vi "write out sonde row.vi"(0 "NI_report in":refnum<class "NI_report.lvclass">, 2 "Columns":i32[](array[numeric]), 3 "Column of Volume":i32, 5 "Sample Sheet Data Row Cluster":T1={"Head\nPressure"=0.0, "Depth"=0.0, "comment "="", "Sonde Data Cluster"={"Cumulative\nVolume (ml)"=100.0, "Specific\nCond (mS)"=2.0, "Dissolved\nOxygen mg/L"=3.0, "pH"=4.0, "ORP"=5.0, "Temp deg C"=26.0, "Salinity"=7.0}, "Aux1"=0.0, "Aux2"=0.0, "Aux3"=0.0} {"Sonde Data Cluster"."Salinity" format="%_3g"; "Sonde Data Cluster"."Temp deg C" format="%_2g"; "Sonde Data Cluster"."ORP" format="%_4g"; "Sonde Data Cluster"."pH" format="%_4g"; "Sonde Data Cluster"."Dissolved\nOxygen mg/L" format="%_4g"; "Sonde Data Cluster"."Specific\nCond (mS)" format="%_4g"; "Sonde Data Cluster"."Cumulative\nVolume (ml)" format="%#_4g"}, 9 "row index":i32, 11 "error in (no error)":errorcluster, 13 "start of last occupied row":cluster{"row":i32, "column":i32}) -> (4 "NI_report out":refnum<class "NI_report.lvclass">, 14 "row index out":i32, 15 "error out":errorcluster)   [LabVIEW 2016]
uses:
  <vilib>/Utility/NIReport.llb/NI_report.lvclass
  sample data row cluster.ctl
  sonde cluster.ctl
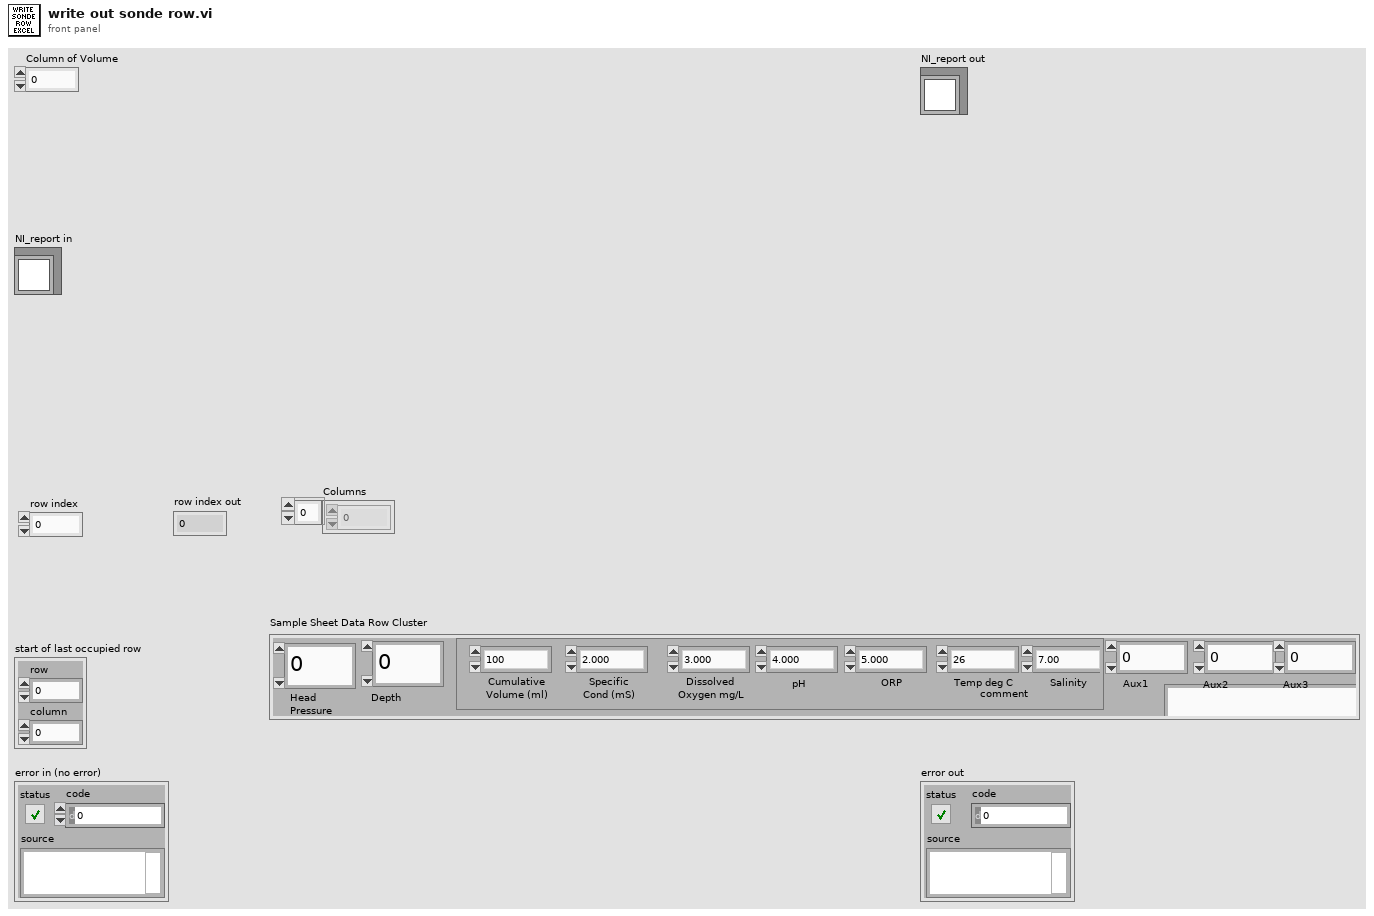
[diagram p1: front panel]
types:
  T1 = typedef "sample data row cluster.ctl" = cluster{"Head\nPressure":dbl, "Depth":dbl, "comment ":string, "Sonde Data Cluster":T2, "Aux1":dbl, "Aux2":dbl, "Aux3":dbl}
  T2 = typedef "sonde cluster.ctl" = cluster{"Cumulative\nVolume (ml)":dbl, "Specific\nCond (mS)":dbl, "Dissolved\nOxygen mg/L":dbl, "pH":dbl, "ORP":dbl, "Temp deg C":dbl, "Salinity":dbl}
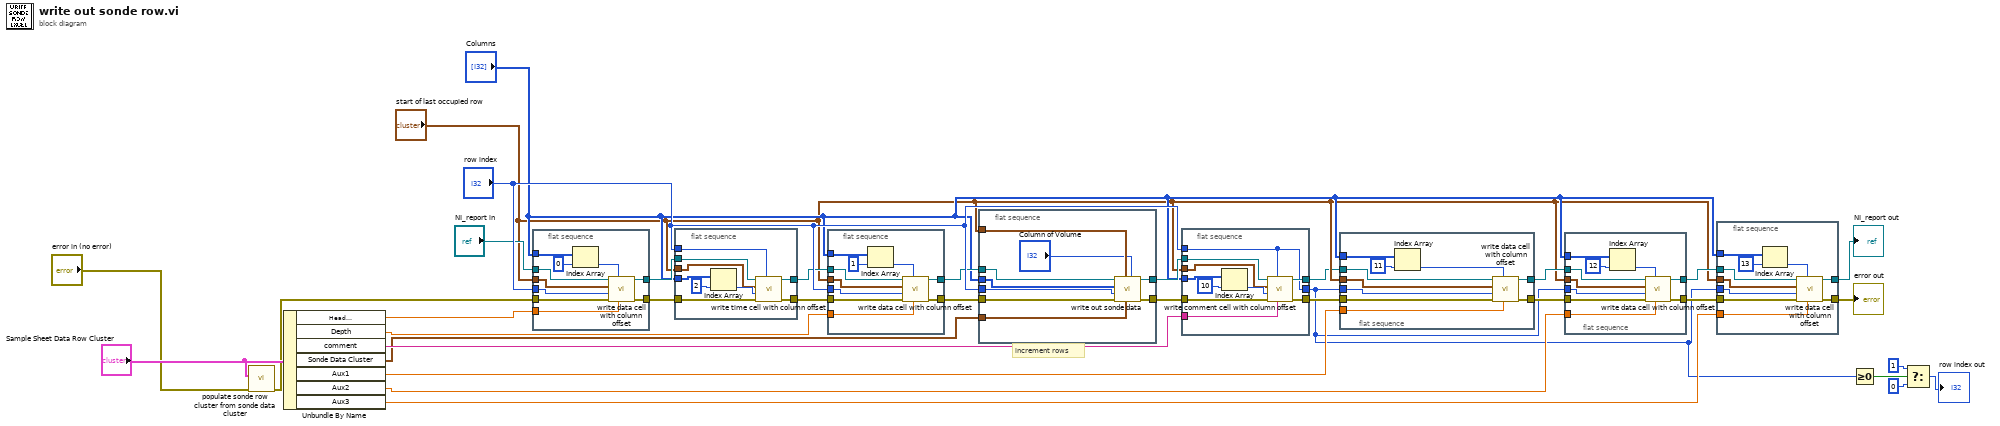
[diagram p0: block diagram]
diagram:
  # "increment rows"
  n1 = call "populate sonde row cluster from sonde data cluster.vi"("error in (no error)"="error in (no error)", "Sample Sheet Data Row Cluster"="Sample Sheet Data Row Cluster") -> ("error out"=w1:errorcluster)  [unwired: 7 in, 2 out]
  n2 = Unbundle By Name("Sample Sheet Data Row Cluster") -> ("Head\nPressure"=w25:dbl, "Depth"=w24:dbl, "comment"=w23:string, "Sonde Data Cluster"=w22:T2, "Aux1"=w16:dbl, "Aux2"=w5:dbl, "Aux3"=w4:dbl)
  n3 = flat-sequence {
    tunnel: "row index" -> [w45]
    tunnel: "start of last occupied row" -> [w44]
    tunnel: [w42] -> w31
    tunnel: [w41] -> w30
    tunnel: "NI_report in" -> [w39]
    tunnel: w1 -> [w38]
    tunnel: "Columns" -> [w37]
    tunnel: w25 -> [w36]
    frame #0 {
      n4 = Index Array(array=w37, index=0) -> (element=w43:i32)
      n5 = call "write data cell with column offset.vi"("Data Input"=w36, "data column"=w43, "error in (no error)"=w38, "row offset"=w45, "start of last occupied row"=w44, "NI_report in"=w39) -> ("error out"=w42:errorcluster, "NI_report out"=w41:refnum<class "NI_report.lvclass">)  [unwired: 4 in]
    }
  }
  n6 = flat-sequence {
    tunnel: "row index" -> [w54]
    tunnel: "start of last occupied row" -> [w51]
    tunnel: w31 -> [w50]
    tunnel: w30 -> [w49]
    tunnel: [w48] -> w29
    tunnel: [w47] -> w28
    tunnel: "Columns" -> [w46]
    frame #0 {
      n7 = Index Array(array=w46, index=2) -> (element=w53:i32)
      n8 = call "write time cell with column offset.vi"("Header offset"=w54, "error in (no error)"=w50, "time column offset"=w53, "start of last occupied row"=w51, "NI_report in"=w49) -> ("error out"=w47:errorcluster, "NI_report out"=w48:refnum<class "NI_report.lvclass">)  [unwired: 5 in]
    }
  }
  n9 = flat-sequence {
    tunnel: "row index" -> [w64]
    tunnel: [w63] -> w34
    tunnel: "start of last occupied row" -> [w62]
    tunnel: w29 -> [w61]
    tunnel: w28 -> [w60]
    tunnel: [w59] -> w27
    tunnel: "Columns" -> [w58]
    tunnel: w24 -> [w55]
    frame #0 {
      n10 = Index Array(array=w58, index=1) -> (element=w56:i32)
      n11 = call "write data cell with column offset.vi"("Data Input"=w55, "data column"=w56, "error in (no error)"=w60, "row offset"=w64, "start of last occupied row"=w62, "NI_report in"=w61) -> ("error out"=w63:errorcluster, "NI_report out"=w59:refnum<class "NI_report.lvclass">)  [unwired: 4 in]
    }
  }
  n12 = flat-sequence {
    tunnel: "row index" -> [w73]
    tunnel: w34 -> [w72]
    tunnel: "Columns" -> [w71]
    tunnel: "start of last occupied row" -> [w70]
    tunnel: [w69] -> w33
    tunnel: [w68] -> w32
    tunnel: w27 -> [w67]
    tunnel: w22 -> [w65]
    frame #0 {
      n13 = call "write out sonde data.vi"("data column offset"="Column of Volume", "Sonde Data Cluster"=w65, "start of last occupied row"=w70, "error in (no error)"=w72, "Row Offset"=w73, "Header data columns"=w71, "NI_report in"=w67) -> ("error out"=w69:errorcluster, "NI_report out"=w68:refnum<class "NI_report.lvclass">)  [unwired: 3 in]
    }
  }
  n14 = flat-sequence {
    tunnel: "row index" -> [w74]
    tunnel: "Columns" -> [w81]
    tunnel: "start of last occupied row" -> [w80]
    tunnel: [w79] -> w7
    tunnel: w33 -> [w78]
    tunnel: [w77] -> w9
    tunnel: w32 -> [w76]
    tunnel: w23 -> [w75]
    tunnel: [w74] -> w3
    frame #0 {
      n15 = Index Array(array=w81, index=10) -> (element=w83:i32)
      n16 = call "write comment cell with column offset.vi"("comment string"=w75, "Row offset"=w74, "error in (no error)"=w78, "comment column offset"=w83, "start of last occupied row"=w80, "NI_report in"=w76) -> ("error out"=w79:errorcluster, "NI_report out"=w77:refnum<class "NI_report.lvclass">)  [unwired: 4 in]
    }
  }
  n17 = flat-sequence {
    tunnel: w3 -> [w93]
    tunnel: [w92] -> w14
    tunnel: "start of last occupied row" -> [w91]
    tunnel: w9 -> [w90]
    tunnel: w7 -> [w89]
    tunnel: [w88] -> w15
    tunnel: "Columns" -> [w87]
    tunnel: w16 -> [w84]
    frame #0 {
      n18 = Index Array(array=w87, index=11) -> (element=w85:i32)
      n19 = call "write data cell with column offset.vi"("Data Input"=w84, "data column"=w85, "error in (no error)"=w89, "row offset"=w93, "start of last occupied row"=w91, "NI_report in"=w90) -> ("error out"=w92:errorcluster, "NI_report out"=w88:refnum<class "NI_report.lvclass">)  [unwired: 4 in]
    }
  }
  n20 = flat-sequence {
    tunnel: w3 -> [w103]
    tunnel: [w102] -> w12
    tunnel: "start of last occupied row" -> [w101]
    tunnel: w15 -> [w100]
    tunnel: w14 -> [w99]
    tunnel: [w98] -> w13
    tunnel: "Columns" -> [w97]
    tunnel: w5 -> [w94]
    frame #0 {
      n21 = Index Array(array=w97, index=12) -> (element=w95:i32)
      n22 = call "write data cell with column offset.vi"("Data Input"=w94, "data column"=w95, "error in (no error)"=w99, "row offset"=w103, "start of last occupied row"=w101, "NI_report in"=w100) -> ("error out"=w102:errorcluster, "NI_report out"=w98:refnum<class "NI_report.lvclass">)  [unwired: 4 in]
    }
  }
  n23 = flat-sequence {
    tunnel: w3 -> [w113]
    tunnel: [w112] -> w6
    tunnel: "start of last occupied row" -> [w111]
    tunnel: w13 -> [w110]
    tunnel: w12 -> [w109]
    tunnel: [w108] -> w8
    tunnel: "Columns" -> [w107]
    tunnel: w4 -> [w104]
    frame #0 {
      n24 = Index Array(array=w107, index=13) -> (element=w105:i32)
      n25 = call "write data cell with column offset.vi"("Data Input"=w104, "data column"=w105, "error in (no error)"=w109, "row offset"=w113, "start of last occupied row"=w111, "NI_report in"=w110) -> ("error out"=w112:errorcluster, "NI_report out"=w108:refnum<class "NI_report.lvclass">)  [unwired: 4 in]
    }
  }
  n26 = Greater Or Equal To 0?(x=w3) -> (x >= 0?=w21:bool)
  n27 = Select(t=1, s=w21, f=0) -> (s? t:f=→"row index out":i32)
  "error out" <- w6
  "NI_report out" <- w8
